vi "Validate State File1.vi"(8 "error in (no error)":errorcluster, 10 "State File ()":string, 11 "VISA resource name":refnum<visa-resource-name>) -> (0 "error out":errorcluster, 2 "Is Valid":bool, 3 "VISA resource name out":refnum<visa-resource-name>)   [LabVIEW 2015, in "Agilent 3446X Series1.lvlib"]
doc: "Checks whether the specified state file exists and contains a valid state file."
uses:
  Agilent 3446X Series1.lvlib
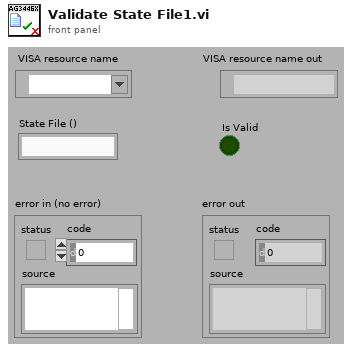
[diagram p1: front panel]
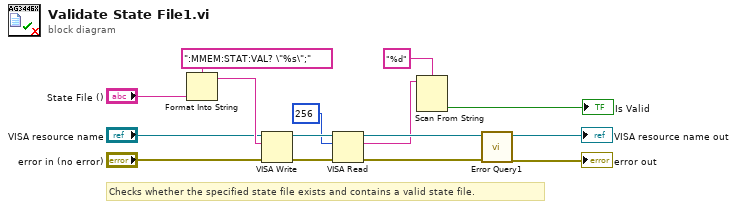
[diagram p0: block diagram]
diagram:
  # "Checks whether the specified state file exists and contains a valid state file."
  n1 = Format Into String(format string=":MMEM:STAT:VAL? \"%s\";", "State File ()") -> (resulting string=w13:string)  [unwired: 2 in, 1 out]
  n2 = VISA Write(VISA resource name="VISA resource name", write buffer=w13, error in (no error)="error in (no error)") -> (VISA resource name out=w8:refnum<visa-resource-name>, error out=w7:errorcluster)  [unwired: 1 out]
  n3 = VISA Read(VISA resource name=w8, byte count=u32 256, error in (no error)=w7) -> (VISA resource name out=w5:refnum<visa-resource-name>, read buffer=w2:string, error out=w4:errorcluster)  [unwired: 1 out]
  n4 = Scan From String(format string="%d", input string=w2) -> (output 1=→"Is Valid":bool)  [unwired: 2 in, 4 out]
  n5 = call "Error Query1.vi"("error in (no error)"=w4, "VISA resource name"=w5) -> ("error out"=→"error out":errorcluster, "VISA resource name out"=→"VISA resource name out":refnum<visa-resource-name>)  [unwired: 8 out]
